vi "Laser Cal.vi"(8 "error in":errorcluster, 11 "P Cal Builder in":refnum<class "P Cal Builder.lvclass">) -> (0 "error out":errorcluster, 1 "SEQ out":refnum<class "SEQ.lvclass">, 2 "Pfinal":dbl, 3 "P Cal Builder out":refnum<class "P Cal Builder.lvclass">)   [LabVIEW 2015, in "P Cal Builder.lvclass"]
doc: "This portion of the builder sets up the integrated area calibration as a function of the pressure. Here we run a sequence of:\n1) Filter ON\n2) Set P\n3) Wait ttot - 30\n4) Turn speaker ON\n5) Wait 5 s\n6) Turn speaker OFF\n7) Wait 25 s\n\nThen, steps 2-7 are repeated until sequence complete. The speaker is required to be on so that the IA is memasured at the right point."
uses:
  P Cal Builder.lvclass
  Reusable/Sequence/SEQ/SEQ.lvclass
  Calibration/Wait/Wait.lvclass
  Sequence/Set Pressure/Set Pressure.lvclass
  Reusable/Sequence/STEPS/LEAVES/String/String STEP.lvclass
  Calibration/Change Spk Pos/Change Speaker Position.lvclass
  Calibration/Change Filter State/Change Filter Position.lvclass
  P Cal Builder.lvclass/P Cal Builder.ctl
  Reusable/Sequence/STEPS/LEAVES/String/String STEP.lvclass/String STEP.ctl
  Reusable/Sequence/STEPS/LEAVES/Double/Switch DBL.lvclass/Switch DBL.ctl
  Calibration/Wait/Wait.lvclass/Wait.ctl
  Reusable/Sequence/STEPS/LEAVES/Double/Switch DBL.lvclass
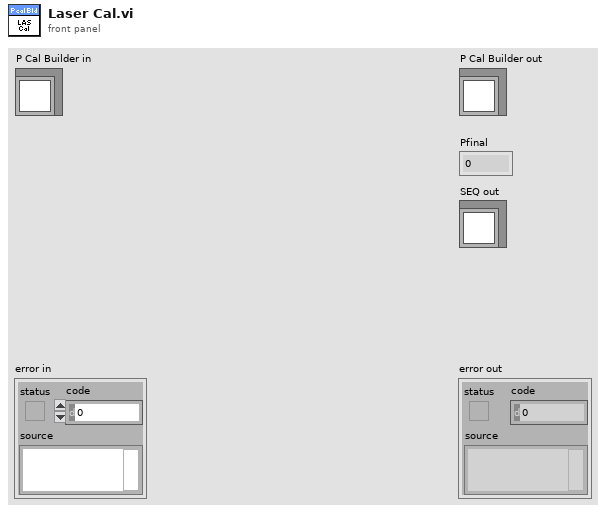
[diagram p1: front panel]
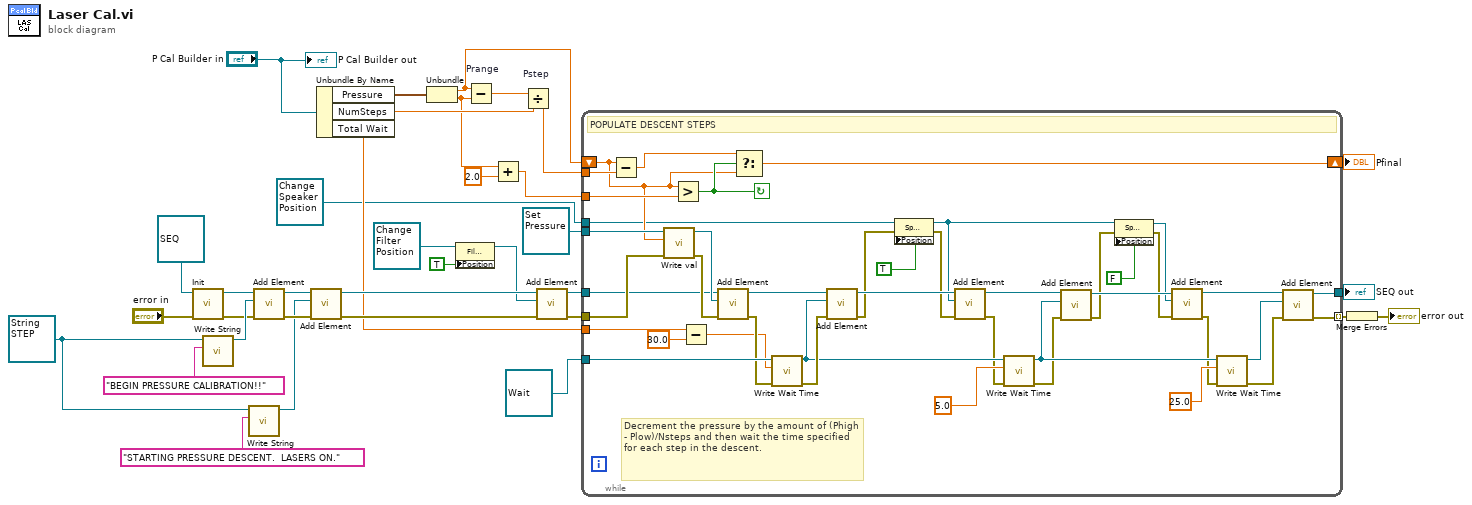
[diagram p0: block diagram]
diagram:
  w29 = refnum<class "String STEP.lvclass"> refnum ("Std MSG STEP")
  n1 = call-dynamic "Init.vi"("error in"="error in", "SEQ in"=refnum<class "SEQ.lvclass"> refnum) -> ("error out"=w11:errorcluster, "SEQ out"=w21:refnum<class "SEQ.lvclass">)  [unwired: 8 in]
  n2 = call "Write String.vi"("String"="BEGIN PRESSURE CALIBRATION!!", "String STEP in"=w29) -> ("String STEP out"=w27:refnum<class "String STEP.lvclass">)  [unwired: 8 in, 1 out]
  n3 = call "Write String.vi"("String"="STARTING PRESSURE DESCENT.  LASERS ON.", "String STEP in"=w29) -> ("String STEP out"=w24:refnum<class "String STEP.lvclass">)  [unwired: 8 in, 1 out]
  n4 = call "Add Element.vi"("error in"=w11, "STEP"=w27, "SEQ in"=w21) -> ("error out"=w25:errorcluster, "SEQ out"=w26:refnum<class "SEQ.lvclass">)  [unwired: 7 in]
  n5 = call "Add Element.vi"("error in"=w25, "STEP"=w24, "SEQ in"=w26) -> ("error out"=w13:errorcluster, "SEQ out"=w20:refnum<class "SEQ.lvclass">)  [unwired: 7 in]
  n6 = Unbundle By Name("P Cal Builder in") -> ("Pressure"=w17:cluster{"Start":dbl, "Final":dbl}, "NumSteps"=w32:dbl, "Total Wait"=w10:dbl)
  n7 = Unbundle(w17) -> ("Start"=w34:dbl, "Final"=w4:dbl)
  n8 = property class="Filter Position"(reference=refnum<class "Change Filter Position.lvclass"> refnum ("Filter Position"), "Position"=TRUE) -> (reference out=w19:refnum<class "Change Filter Position.lvclass">)  [unwired: 1 in, 1 out]
  n9 = Subtract "Prange"(x=w34, y=w4) -> (x-y=w33:dbl)
  n10 = Add(x=w4, y=2.0) -> (x+y=w2:dbl)
  n11 = Divide "Pstep"(x=w33, y=w32) -> (x/y=w31:dbl)
  n12 = call "Add Element.vi"("error in"=w13, "STEP"=w19, "SEQ in"=w20) -> ("error out"=w12:errorcluster, "SEQ out"=w16:refnum<class "SEQ.lvclass">)  [unwired: 7 in]
  n13 = while {
    tunnel: refnum<class "Set Pressure.lvclass"> refnum ("Set Pressure Step") -> [w75]
    tunnel: w2 -> [w76]
    tunnel: w31 -> [w77]
    shift-right: [w64] -> w5
    shift-left: w34 -> [w65]
    tunnel: refnum<class "Wait.lvclass"> refnum ("Wait") -> [w72]
    tunnel: [w45] -> w6
    tunnel: [w44] -> w8 mode=indexing
    tunnel: w12 -> [w68]
    tunnel: w10 -> [w62]
    tunnel: w16 -> [w63]
    tunnel: refnum<class "Change Speaker Position.lvclass"> refnum ("Spk Pos") -> [w57]
    stop <- w67 continue-if-true
    # "Decrement the pressure by the amount of (Phigh - Plow)/Nsteps and then wait the time specified for each step in the descent."
    # "POPULATE DESCENT STEPS"
    n14 = Subtract(x=w65, y=w77) -> (x-y=w66:dbl)
    n15 = call "Write val.vi"("error in (no error)"=w68, "val"=w65, "Switch DBL in"=w75) -> ("error out"=w74:errorcluster, "Switch DBL out"=w73:refnum<class "Set Pressure.lvclass">)  [unwired: 7 in]
    n16 = Greater?(x=w65, y=w76) -> (0:w67:bool)
    n17 = Subtract(x=w62, y=30.0) -> (x-y=w60:dbl)
    n18 = call "Add Element.vi"("error in"=w74, "STEP"=w73, "SEQ in"=w63) -> ("error out"=w70:errorcluster, "SEQ out"=w71:refnum<class "SEQ.lvclass">)  [unwired: 7 in]
    n19 = Select(t=w66, s=w67, f=w65) -> (s? t:f=w64:dbl)
    n20 = call "Write Wait Time.vi"("error in (no error)"=w70, "Wait Time"=w60, "Wait in"=w72) -> ("error out"=w69:errorcluster, "Wait out"=w55:refnum<class "Wait.lvclass">)  [unwired: 7 in]
    n21 = call "Add Element.vi"("error in"=w69, "STEP"=w55, "SEQ in"=w71) -> ("error out"=w43:errorcluster, "SEQ out"=w59:refnum<class "SEQ.lvclass">)  [unwired: 7 in]
    n22 = property class="Spk Pos"(reference=w57, error in=w43, "Position"=TRUE) -> (reference out=w53:refnum<class "Change Speaker Position.lvclass">, error out=w42:errorcluster)
    n23 = call "Add Element.vi"("error in"=w42, "STEP"=w53, "SEQ in"=w59) -> ("error out"=w41:errorcluster, "SEQ out"=w56:refnum<class "SEQ.lvclass">)  [unwired: 7 in]
    n24 = call "Write Wait Time.vi"("error in (no error)"=w41, "Wait Time"=5.0, "Wait in"=w55) -> ("error out"=w40:errorcluster, "Wait out"=w48:refnum<class "Wait.lvclass">)  [unwired: 7 in]
    n25 = call "Add Element.vi"("error in"=w40, "STEP"=w48, "SEQ in"=w56) -> ("error out"=w39:errorcluster, "SEQ out"=w51:refnum<class "SEQ.lvclass">)  [unwired: 7 in]
    n26 = property class="Spk Pos"(reference=w53, error in=w39, "Position"=FALSE) -> (reference out=w50:refnum<class "Change Speaker Position.lvclass">, error out=w38:errorcluster)
    n27 = call "Add Element.vi"("error in"=w38, "STEP"=w50, "SEQ in"=w51) -> ("error out"=w37:errorcluster, "SEQ out"=w49:refnum<class "SEQ.lvclass">)  [unwired: 7 in]
    n28 = call "Write Wait Time.vi"("error in (no error)"=w37, "Wait Time"=25.0, "Wait in"=w48) -> ("error out"=w36:errorcluster, "Wait out"=w46:refnum<class "Wait.lvclass">)  [unwired: 7 in]
    n29 = call "Add Element.vi"("error in"=w36, "STEP"=w46, "SEQ in"=w49) -> ("error out"=w44:errorcluster, "SEQ out"=w45:refnum<class "SEQ.lvclass">)  [unwired: 7 in]
  }
  "SEQ out" <- w6
  "Pfinal" <- w5
  n30 = Merge Errors(w8) -> (→"error out":errorcluster)
  "P Cal Builder out" <- "P Cal Builder in"
